vi "CloseHardware.vi"(8 "error in (no error)":errorcluster, 11 "XPS-RLD in":refnum<class "XPS-RLD.lvclass">) -> (0 "error out":errorcluster)   [LabVIEW 2020, in "XPS-RLD.lvclass"]
uses:
  XPS-RLD/XPS-RLD.lvclass
  XPS-RLD/XPS-RLD.lvclass/XPS-RLD.ctl
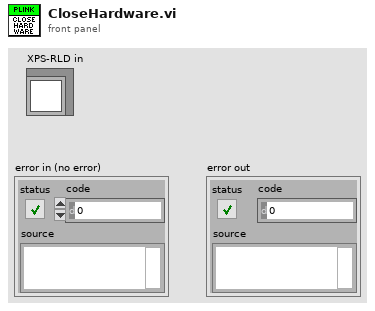
[diagram p1: front panel]
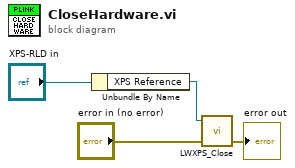
[diagram p0: block diagram]
diagram:
  n1 = Unbundle By Name("XPS-RLD in") -> ("XPS Reference"=w2:refnum<k24>)
  n2 = call "LWXPS_Close.vi"("LabVIEW error IN"="error in (no error)", "CommandInterfaceXPS.XPS"=w2) -> ("LabVIEW error OUT"=→"error out":errorcluster)  [unwired: 2 in, 1 out]
